vi "AO master control_v2.vi"() -> ()   [LabVIEW 2018]
uses:
  Casao LabVIEW SDK 1.0.5/Haso/Data Haso/Wavefront parameters.ctl
  Casao LabVIEW SDK 1.0.5/Casao/Casao/Casao.ctl
  Casao LabVIEW SDK 1.0.5/Drivers_DPhaseModul/PhaseModul.ctl
  Casao LabVIEW SDK 1.0.5/Casao/CasaoMatrix/CasaoMatrix.ctl
  Casao LabVIEW SDK 1.0.5/Haso/Haso/Haso.ctl
  Casao LabVIEW SDK 1.0.5/Haso/Camera/Camera.ctl
  <vilib>/Utility/error.llb/DialogType.ctl
  Casao LabVIEW SDK 1.0.5/Casao/Casao/Loop prefs.ctl
  Casao LabVIEW SDK 1.0.5/Haso/Data Haso/DataHaso.ctl
  <vilib>/DAQmx/write.llb/DAQmx Write (Digital Bool 1Line 1Point).vi
  <vilib>/Utility/file.llb/Read From Spreadsheet File (DBL).vi
  <vilib>/DAQmx/create/channels.llb/DAQmx Create Channel (DO-Digital Output).vi
  <vilib>/DAQmx/miscellaneous.llb/DAQmx Fill In Error Info.vi
  <vilib>/Utility/file.llb/Write To Spreadsheet File (DBL).vi
panel:
  in  "Phase command 3":path=path "D:/SystemAlignment/system_aberration_20191029.dat"
  in  "Phase command 2":path=path "D:/SystemAlignment/100nm correction.dat"
  in  "Phase command 1":path=path "D:/SystemAlignment/FLAT_MIRAO_0225_01.dat"
  in  "Phase command 0":path=path "D:/SystemAlignment/system_aberration_20191029.dat"
  out "error out 3":errorcluster
  out "error out 2":errorcluster
  out "error out 4":errorcluster
  out "error out":errorcluster
  in  "Control Panel":T1(tab)
  in  "Haso Serial #":T2=7364
  out "Camera Index":T3
  out "Haso Index":T2
  out "Casao Matrix Index":T4
  out "Initialization error":errorcluster
  in  "Matrix Initial":path=path "D:/Data/CM_20191031.aomc"
  out "Mirror Index":T5
  in  "DM Initial":path=path "D:/SystemAlignment/system_aberration_20191029.dat"
  out "Casao Index":T6
  in  "Stage Port":refnum<visa-resource-name>="COM5"
  in  "Flip Mirror Port":tag="Dev1/ao5"
  in  "EMCCD trigger port":tag="Dev1/port0/line0"
  in  "EMCCD fire port":tag="/Dev1/PFI0"
  in  "Laser 2P shutter port":tag="Dev1/port0/line1"
  in  "Laser 488 shutter port":tag="Dev1/port0/line3"
  in  "baud rate (9600)":u32=9600
  in  "Mirao Parameters":path=path "C:/Program Files (x86)/Imagine Optic/Configuration Files/mirao 52-e 0225.xml"
  in  "Haso Exposure (s) Initial":dbl=0.5
  in  "Update DM":bool
  in  "right":bool
  in  "left":bool
  in  "front":bool
  in  "back":bool
  in  "XY step (10=1um)":u16=50
  in  "down":bool
  in  "up":bool
  in  "Z step (10=1um)":dbl=2.0
  in  "stop adjustment":bool
  in  "WideField 488":bool
  in  "Flip Mirror":sgl(ring)=-5.0 items=["EMCCD Camera"=-5, "Wavefront sensor"=1]
  out "Numeric status":dbl
  in  "Two photon":bool
  in  "Offset path":path=path "D:/SystemAlignment/system_aberration_20191029.dat"
  in  "Matrix path":path=path "D:/Data/CM_20191031.aomc"
  in  "Acquisition Mode":T7(ring) caption="Acquistion Mode"
  out "Wavefront after correction":dbl[][](graph) caption="Wavefront"
  out "Wavefront before correction":dbl[][](graph) caption="Wavefront"
  out "output path":path
  in  "Correction":bool
  in  "Slices #":dbl=2.0
  in  "Average Frame #":dbl=1.0
  in  "Offset path 2":path=path "D:/Data/system_aberration_20191029.dat"
  in  "Matrix path 2":path=path "D:/Data/CM_20191031.aomc"
  out "Model Coefficients (µm) before":sgl[](array[numeric])
  in  "Iteration #":u16(ring)=1 items=["1"=1, "2"=2, "3"=3, "4"=4, "5"=5]
  in  "AoExp Time":dbl(ring)=0.5 items=["0.2s"=0.2, "0.5s"=0.5, "1.0s"=1.0, "1.5s"=1.5]
  in  "stop":bool
  out "Camera image":u32[][](graph)
  out "before correction":T8
  out "after correction":T8
  in  "Step size(um)":dbl
  in  "ImExp Time (s)":dbl(ring)=0.1 items=["0.05"=0.05, "0.1"=0.1, "0.2"=0.2, "0.5"=0.5, "1.0"=1.0, "4.0"=4.0, "8.0"=8.0]
  out "Slice now":dbl
  in  "Filter y tilt":bool=TRUE
  in  "Filter x tilt":bool=TRUE
  in  "Curvature filter":bool=TRUE
  out "RMS":dbl
  out "PV":dbl
  out "PV":dbl
  out "RMS":dbl
  in  "Filter y tilt":bool=TRUE
  in  "Filter x tilt":bool=TRUE
  in  "Curvature filter":bool=TRUE
  out "Model Coefficients (µm) after":sgl[](array[numeric])
  out "Shutdown error":errorcluster
  in  "Control Mode":T9(ring)=enum."Parameter Adjustment"
  # "Port connections"
  # "Casao Initialization"
  # "Casao Status"
  # "Sample Stage"
  # "WF switch"
  # "EMCCD: -5"
  # "Wavefront Sensor: 1"
  # "Laser Shutter"
  # "Deformable Mirror"
  # "Wavefront Sensor"
  # "AO correction (Casao)"
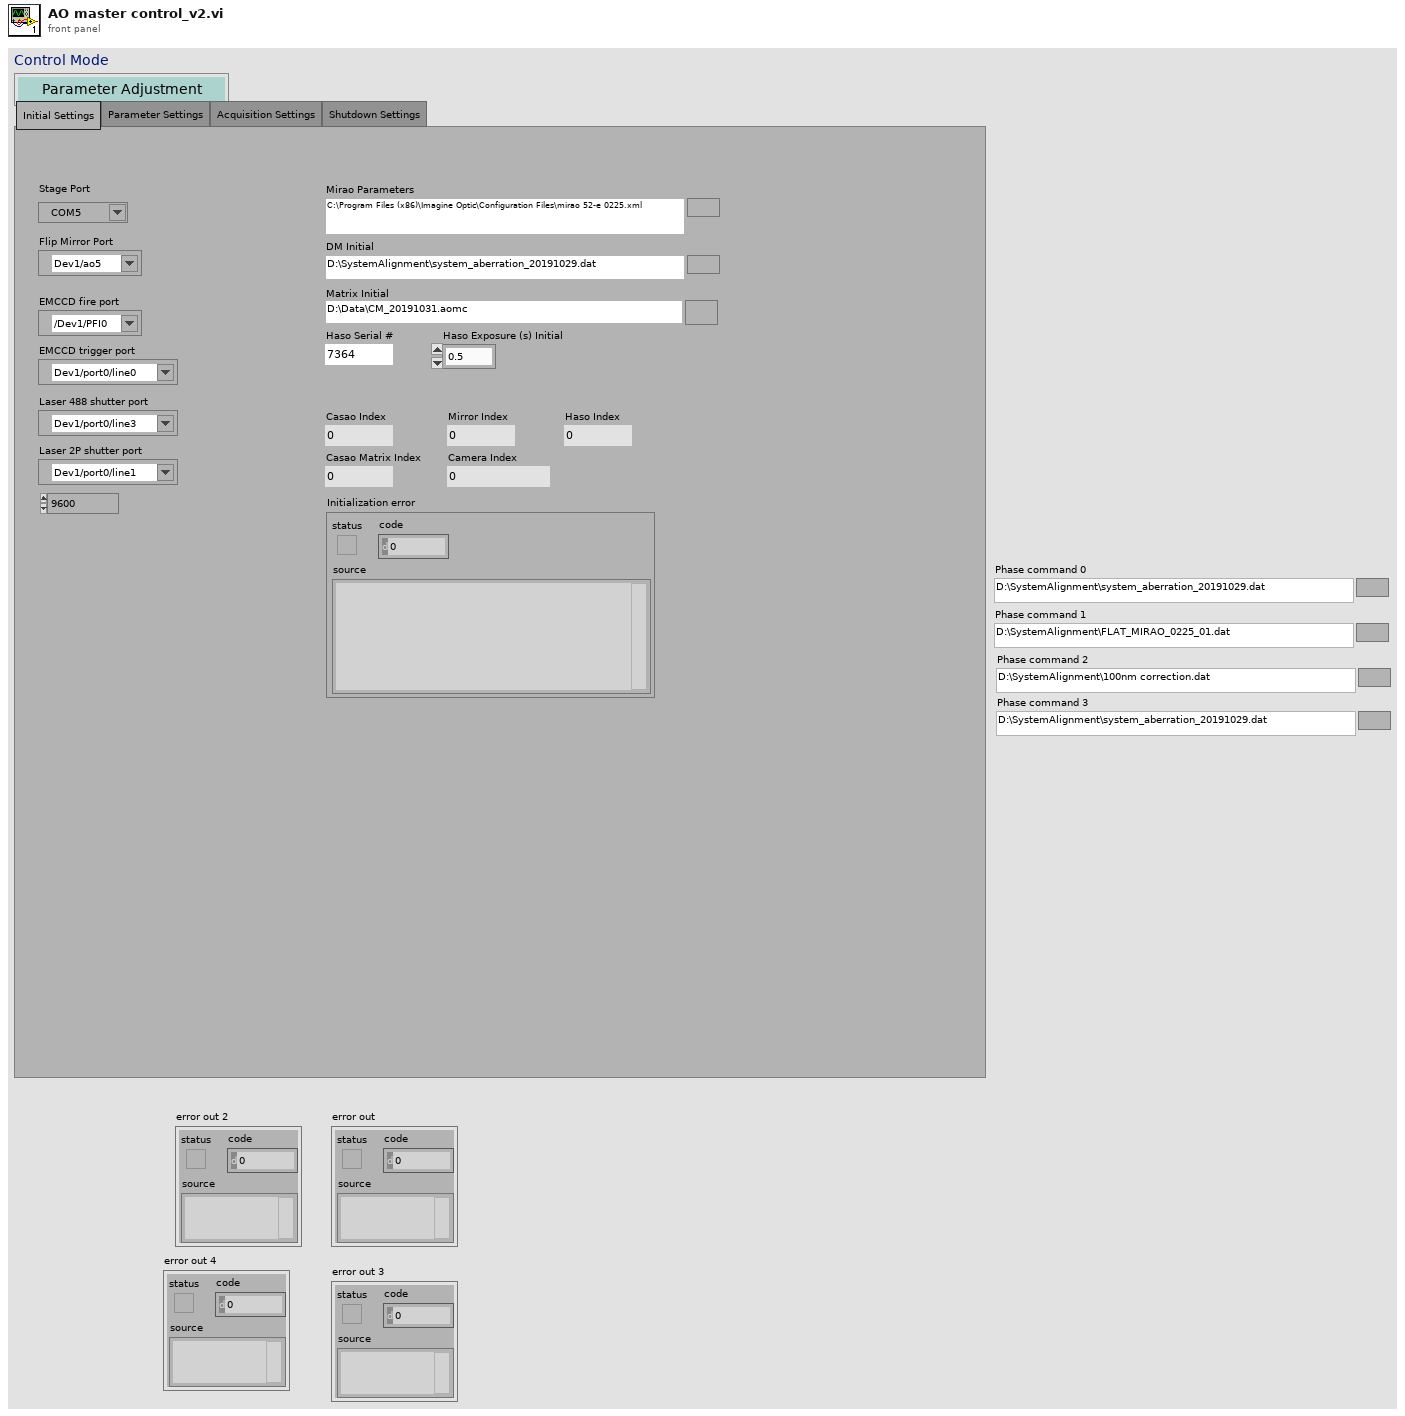
[diagram p1: front panel]
types:
  T1 = enum32{"Initial Settings", "Parameter Settings", "Acquisition Settings", "Shutdown Settings"}
  T2 = typedef "Haso.ctl" = i32
  T3 = typedef "Camera.ctl" = i32
  T4 = typedef "CasaoMatrix.ctl" = i32
  T5 = typedef "PhaseModul.ctl" = i32
  T6 = typedef "Casao.ctl" = i32
  T7 = enum16{"Wide Field", "Wide Field (Phase diversity)", "Two photon"}
  T8 = typedef "Wavefront parameters.ctl" = cluster{"X Tilt (mrad)":sgl, "Y Tilt (mrad)":sgl, "Radius of curvature (mm)":sgl, "X focal point position (mm)":sgl, "Y focal point position (mm)":sgl, "Astigmatism angle (rad)":sgl, "Sagittal focal length (mm)":sgl, "Tangential focal length (mm)":sgl}
  T9 = enum16{"Initialization", "Parameter Adjustment", "Acquisition", "Shut Down"}
  T10 = typedef "Loop prefs.ctl" = cluster{"Filter tilt on measurement (closed loop)":bool, "Correction gain (closed loop)":sgl, "Limit of subapertures off in CGP (%)":sgl, "Limit of saturated actuators (%)":sgl}
  T11 = cluster{"Filtre tilt X":bool, "Filtre tilt Y":bool, "Filtre courbure":bool}
  T12 = typedef "DataHaso.ctl" = i32
  T13 = cluster{"Measurement":T12, "Target":T12, "Manual target":T12}
  T14 = cluster{"Target for tilt":T12, "Target for focus":T12, "Target for all other aberrations":T12}
  T15 = typedef "Camera preferences.ctl" = cluster{"Exposure duration (µs)":u32, "Exposure duration specified (µs)":u32, "Number of summed images":u32, "Trigger type":enum16{"Internal", "TTL", "Software"}, "Trigger event":enum16{"falling", "rising"}, "Remove background image":bool, "Background image":T16, "Path to background image":string, "Auto exposure":bool, "Auto exposure target (%)":sgl, "Auto exposure tolerance (%)":sgl, "Timeout delay (ms)":u32, "Delay after trigger (µs)":i32}
  T16 = typedef "Image Compat.ctl" = cluster{"Signed/unsigned":bool, "Number of bits":T17, "Internal object id":i32, "Internal data id":i32}
  T17 = typedef "Data alignment enum.ctl" = enum16{"8", "16", "32"}
  T18 = typedef "DialogType.ctl" = u16
  T19 = typedef "Reconstruction prefs.ctl" = cluster{"Reconstruction type":enum16{"Modal", "Zonal"}, "Polynomial type":enum16{"Zernike", "Legendre"}, "Modal reconstruction prefs":T20, "Zonal reconstruction prefs":T23}
  T20 = typedef "Modal reconstruction prefs.ctl" = cluster{"Number of coefficients":u32, "Filtered coefficients":u32[], "RMS Zernike normalization":bool, "Matrix inversion method":u16, "Add zonal residual to modal fit ":bool, "Detection prefs":T21}
  T21 = typedef "PupilDetectionPrefs.ctl" = cluster{"Automatic pupil detection":bool, "Central occultation pupil":bool, "Semi-automatic pupil detection (find radius)":bool, "Semi-automatic pupil detection (find center)":bool, "Automatic pupil detection mode":enum16{"Contained", "Containing"}, "Start coordinates":cluster{"Pupil center (Zernike)":T22, "Pupil radius (Zernike)":sgl, "Pupil center (Legendre)":T22, "Pupil halfsize (Legendre)":T22}}
  T22 = typedef "Point2Df.ctl" = cluster{"X":sgl, "Y":sgl}
  T23 = typedef "Zonal reconstruction prefs.ctl" = cluster{"Number of weak iterations":u16, "Number of max iterations":u32, "Residual limit":sgl}
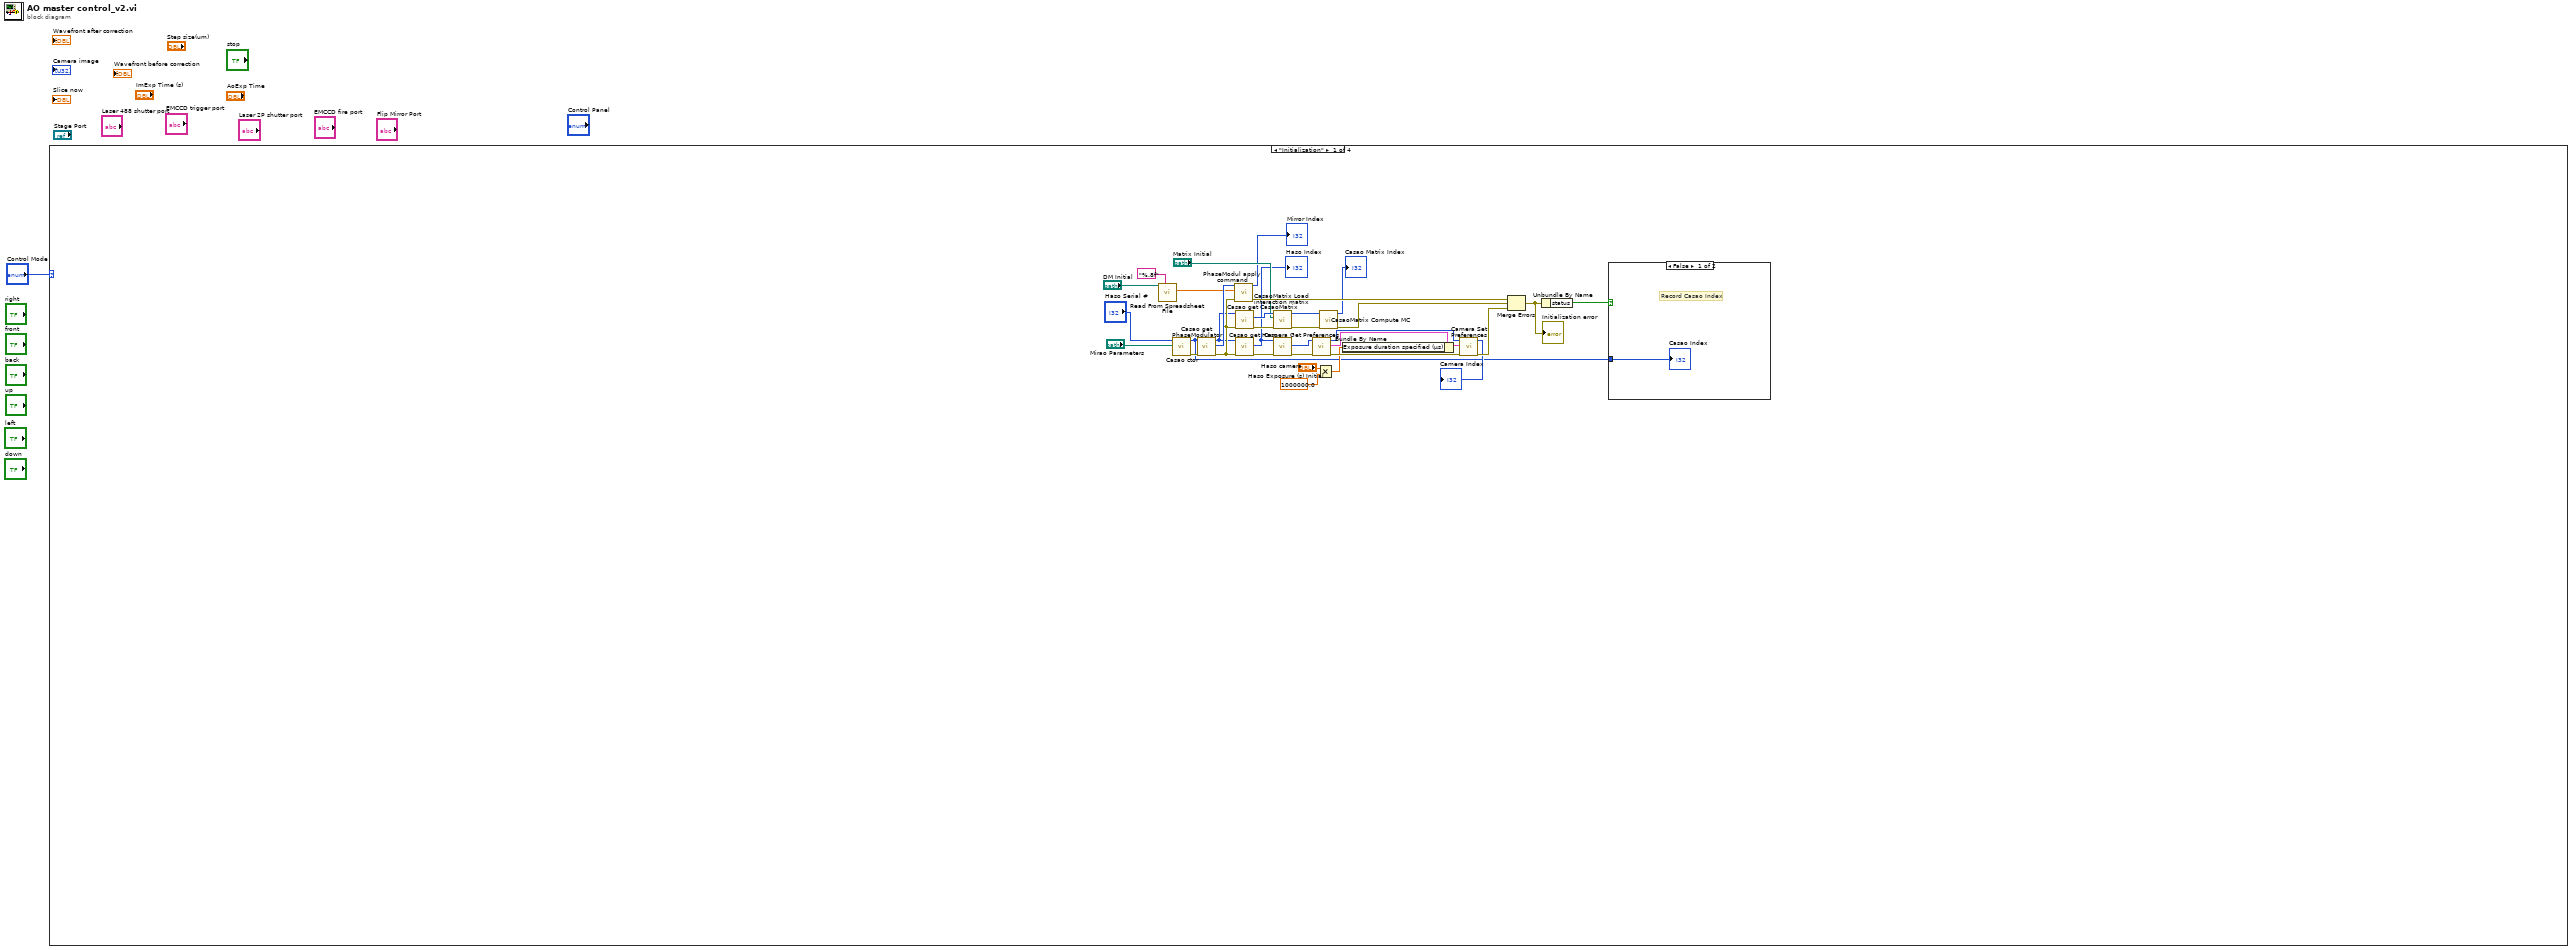
[diagram p0: block diagram]
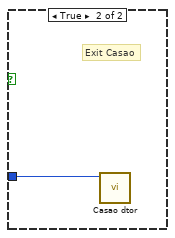
[diagram p2: hidden frame]
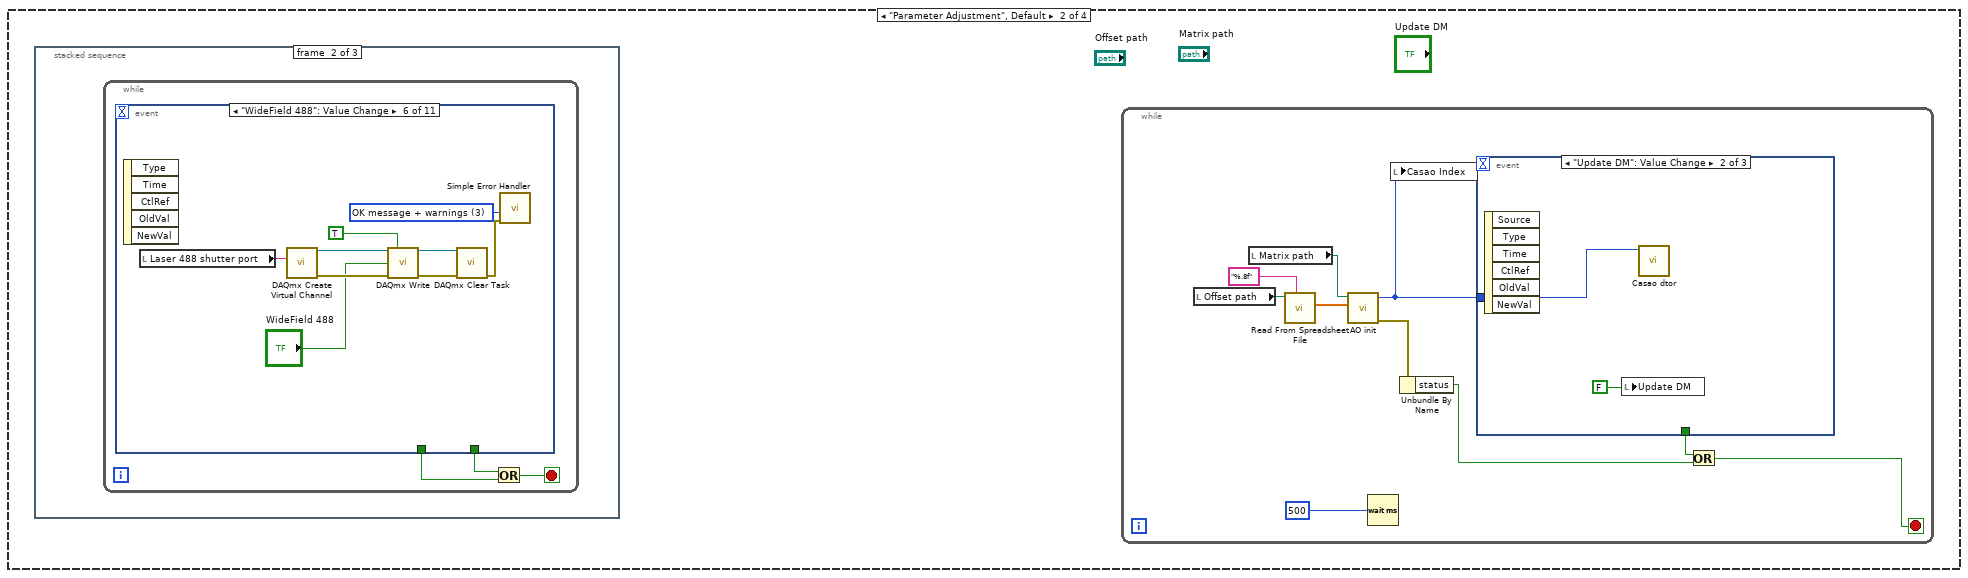
[diagram p3: hidden frame]
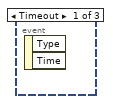
[diagram p4: hidden frame]
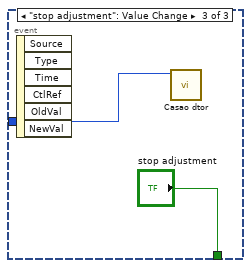
[diagram p5: hidden frame]
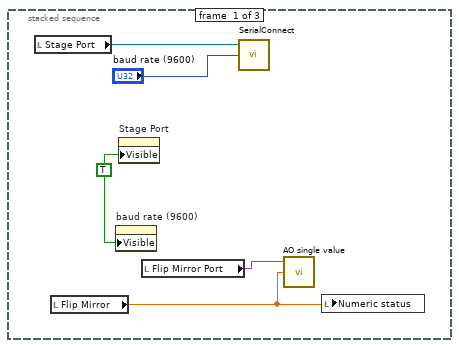
[diagram p6: hidden frame]
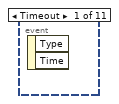
[diagram p7: hidden frame]
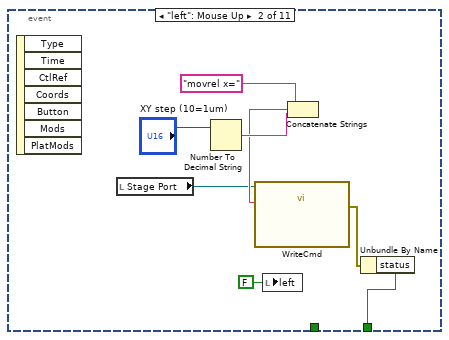
[diagram p8: hidden frame]
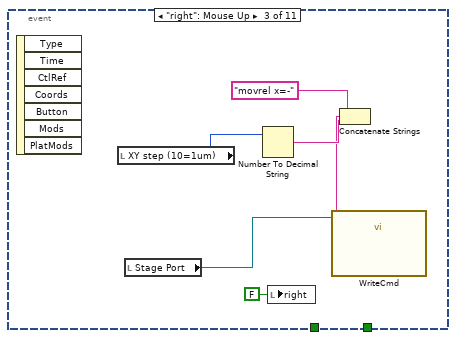
[diagram p9: hidden frame]
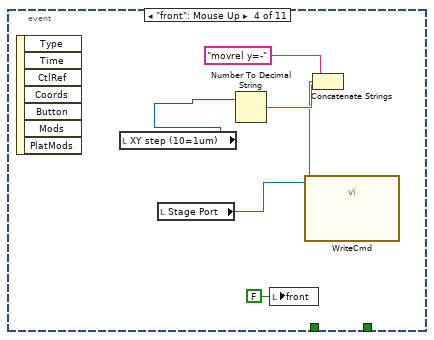
[diagram p10: hidden frame]
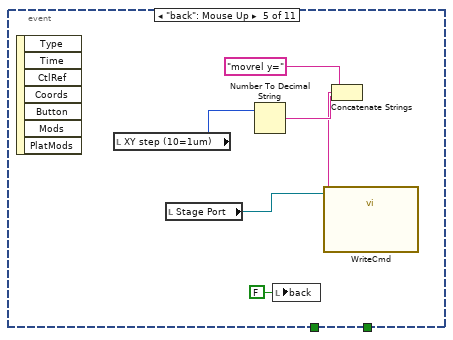
[diagram p11: hidden frame]
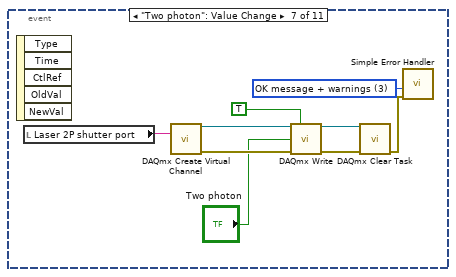
[diagram p12: hidden frame]
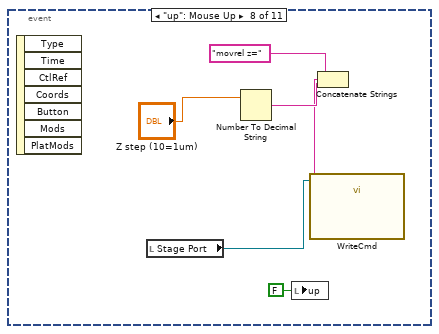
[diagram p13: hidden frame]
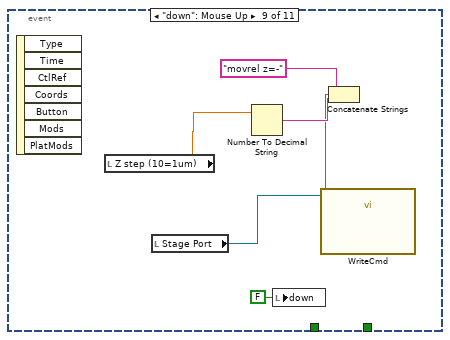
[diagram p14: hidden frame]
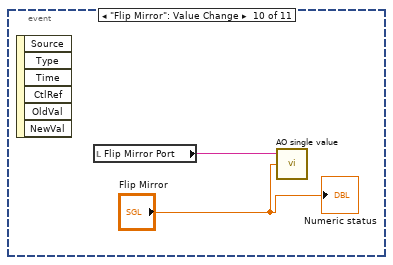
[diagram p15: hidden frame]
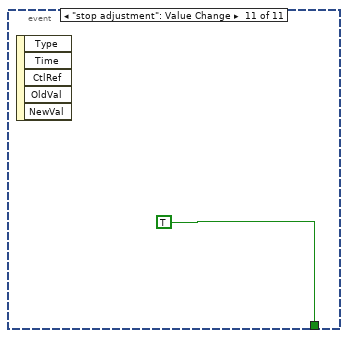
[diagram p16: hidden frame]
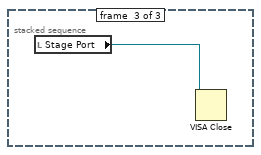
[diagram p17: hidden frame]
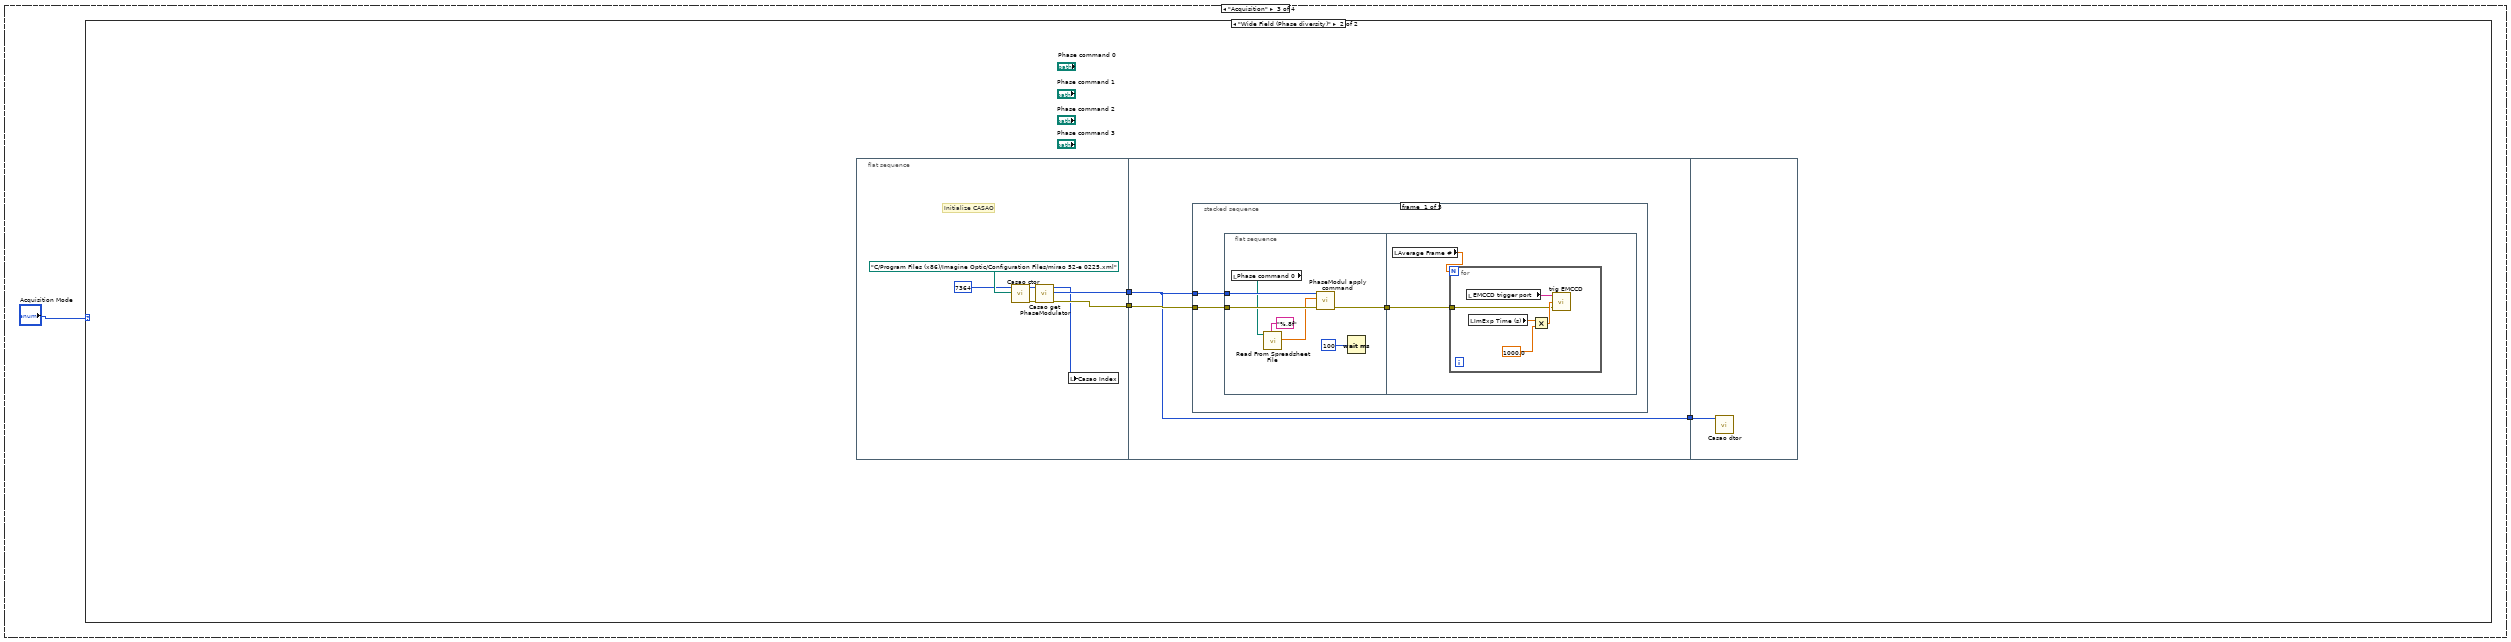
[diagram p18: hidden frame]
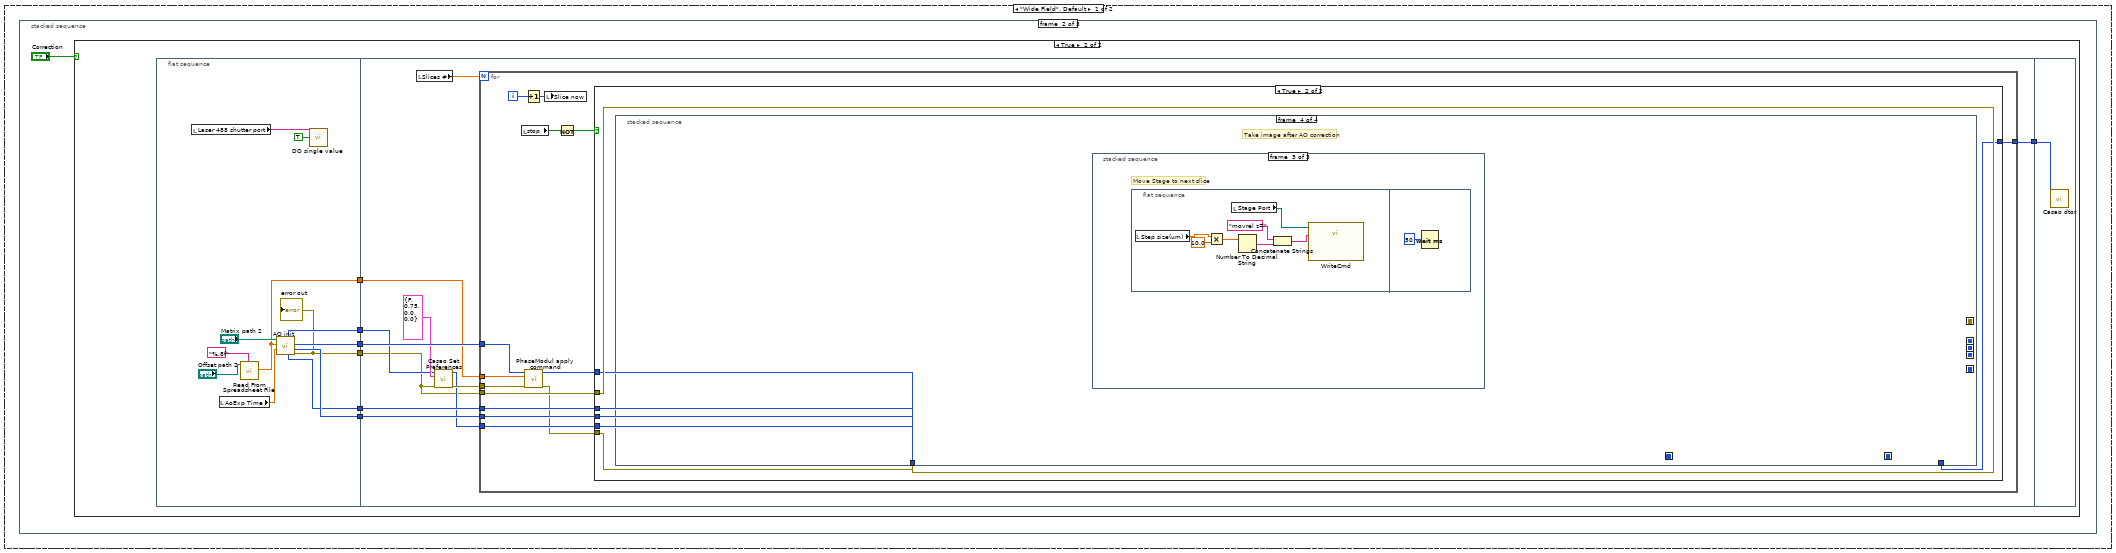
[diagram p19: hidden frame]
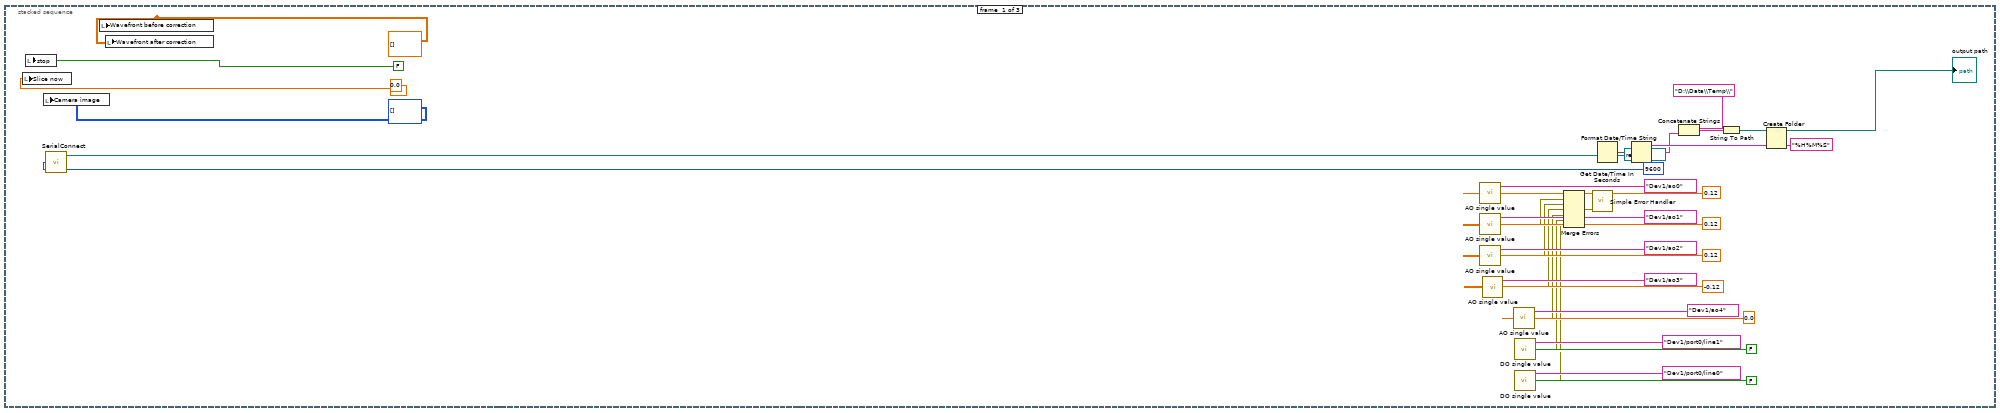
[diagram p20: hidden frame]
diagram:
  n1 = case shown="\"Initialization\"" "Control Mode" {
    frame "Initialization" {
      n2 = call-poly <vilib>:"Read From Spreadsheet File.vi"("format (%.3f)"="%.8f", "file path (dialog if empty)"="DM Initial") -> ("first row"=w10:dbl[])  [unwired: 5 in, 4 out]
      n3 = call "Casao ctor.vi"("Mirror config file path"="Mirao Parameters", "Haso serial number"="Haso Serial #") -> ("error out"=w19:errorcluster, "Casao"=w2:T6)  [unwired: 6 in]
      n4 = call "Casao get PhaseModulator.vi"("error in (no error)"=w19, "Casao"=w2) -> ("error out"=w21:errorcluster, "Mirrror"=w20:T5, "Casao (dup)"=w17:T6)  [unwired: 3 in]
      n5 = call "PhaseModul apply command.vi"("error in (no error)"=w21, "Commands in"=w10, "Mirror"=w20) -> ("error out"=w18:errorcluster, "Mirror (dup)"=→"Mirror Index":T5)  [unwired: 2 in, 1 out]
      n6 = call "Casao get CasaoMatrix.vi"("error in (no error)"=w21, "Casao"=w17) -> ("error out"=w32:errorcluster, "Casao matrix"=w31:T4)  [unwired: 3 in, 1 out]
      n7 = call "Casao get Haso.vi"("error in (no error)"=w21, "Casao"=w17) -> ("error out"=w28:errorcluster, "Haso"=w6:T2)  [unwired: 3 in, 1 out]
      "Haso Index" <- w6
      n8 = call "CasaoMatrix Load interaction matrix.vi"("error in (no error)"=w32, "Path"="Matrix Initial", "Casao matrix"=w31) -> ("error out"=w30:errorcluster, "Casao matrix (dup)"=w29:T4)  [unwired: 1 in, 2 out]
      n9 = call "Haso camera.vi"("error in (no error)"=w28, "Haso"=w6) -> ("error out"=w27:errorcluster, "camera"=w26:T3)  [unwired: 3 in, 1 out]
      n10 = call "Camera Get Preferences.vi"("error in (no error)"=w27, "Camera"=w26) -> ("error out"=w25:errorcluster, "Camera Preferences"=w24:T15, "Camera (dup)"=w23:T3)  [unwired: 3 in]
      n11 = Multiply(x="Haso Exposure (s) Initial", y=1000000.0) -> (x*y=w11:dbl)
      n12 = call "CasaoMatrix Compute MC.vi"("error in (no error)"=w30, "Casao Matrix"=w29) -> ("error out"=w9:errorcluster, "Casao Matrix (dup)"=→"Casao Matrix Index":T4)  [unwired: 4 in]
      n13 = Bundle By Name(cluster=w24, "Exposure duration specified (µs)"=w11) -> (w22:T15)
      n14 = call "Camera Set Preferences.vi"("error in (no error)"=w25, "Camera Preferences"=w22, "Camera"=w23) -> ("error out"=w16:errorcluster, "Camera (dup)"=→"Camera Index":T3)  [unwired: 3 in]
      n15 = Merge Errors(w18, w9, w16) -> (w3:errorcluster)
      "Initialization error" <- w3
      n16 = Unbundle By Name(w3) -> ("status"=w33:bool)
      n17 = case shown="False" w33 {
        tunnel: w2 -> [w36 w37]
        frame False {
          # "Record Casao Index"
          "Casao Index" <- w36
        }
        frame True {
          # "Exit Casao"
          n18 = call "Casao dtor.vi"("Casao"=w37) -> ()  [unwired: 6 in, 1 out]
        }
      }
    }
    frame "Parameter Adjustment", Default {
      n19 = stacked-sequence {
        frame #0 {
          w55 = TRUE ("Visible")
          n20 = local read "Stage Port"() -> (w53:refnum<visa-resource-name>)
          n21 = local read "Flip Mirror"() -> (w54:sgl)
          n22 = property on="baud rate (9600)" class="DigNum (strict)"("Visible"=w55) -> ()  [unwired: 2 in, 2 out]
          n23 = property on="Stage Port" class="VISAName"("Visible"=w55) -> ()  [unwired: 2 in, 2 out]
          n24 = local read "Flip Mirror Port"() -> (w52:tag)
          n25 = call "SerialConnect.vi"("baud rate (9600)"="baud rate (9600)", "VISA resource name"=w53) -> ()  [unwired: 1 in, 3 out]
          n26 = call "AO single value.vi"("data"=w54, "physical channels"=w52) -> ()  [unwired: 1 in, 1 out]
          n27 = local write "Numeric status"(w54) -> ()
        }
        frame #1 {
          n28 = while {
            stop <- w59 stop-if-true
            n29 = event shown="[5] \"WideField 488\": Value Change" {
              selector: _ -> [_ _ _ _ _ _ _ _ _ _ _]
              dyn-events: _ -> [_ _ _ _ _ _ _ _ _ _ _]
              timeout: _ -> [_ _ _ _ _ _ _ _ _ _ _]
              tunnel: [_ _ _ _ _ _ _ _ _ _ TRUE] -> w58
              tunnel: [_ w60 _ _ _ _ _ _ _ _ _] -> w57
              event Timeout {
                n30 = event-data() -> ()  [unwired: 1 in, 2 out]
              }
              event "left": Mouse Up {
                n31 = event-data() -> ()  [unwired: 1 in, 7 out]
                n32 = local read "Stage Port"() -> (w63:refnum<visa-resource-name>)
                n33 = Number To Decimal String(number="XY step (10=1um)") -> (decimal integer string=w65:string)  [unwired: 1 in]
                n34 = local write "left"(FALSE ("left")) -> ()
                n35 = Concatenate Strings("movrel x=", w65) -> (w64:string)
                n36 = call "WriteCmd.vi"("Command"=w64, "VISA resource name"=w63) -> ("error"=w61:errorcluster)  [unwired: 1 in]
                n37 = Unbundle By Name(w61) -> ("status"=w60:bool)
              }
              event "right": Mouse Up {
                n38 = event-data() -> ()  [unwired: 1 in, 7 out]
                n39 = local read "XY step (10=1um)"() -> (w69:u16)
                n40 = local read "Stage Port"() -> (w68:refnum<visa-resource-name>)
                n41 = Number To Decimal String(number=w69) -> (decimal integer string=w72:string)  [unwired: 1 in]
                n42 = local write "right"(FALSE ("right")) -> ()
                n43 = Concatenate Strings("movrel x=-", w72) -> (w71:string)
                n44 = call "WriteCmd.vi"("Command"=w71, "VISA resource name"=w68) -> ()  [unwired: 1 in, 1 out]
              }
              event "front": Mouse Up {
                n45 = event-data() -> ()  [unwired: 1 in, 7 out]
                n46 = local read "XY step (10=1um)"() -> (w74:u16)
                n47 = local read "Stage Port"() -> (w76:refnum<visa-resource-name>)
                n48 = Number To Decimal String(number=w74) -> (decimal integer string=w78:string)  [unwired: 1 in]
                n49 = local write "front"(FALSE ("front")) -> ()
                n50 = Concatenate Strings("movrel y=-", w78) -> (w77:string)
                n51 = call "WriteCmd.vi"("Command"=w77, "VISA resource name"=w76) -> ()  [unwired: 1 in, 1 out]
              }
              event "back": Mouse Up {
                n52 = event-data() -> ()  [unwired: 1 in, 7 out]
                n53 = local read "XY step (10=1um)"() -> (w80:u16)
                n54 = local read "Stage Port"() -> (w82:refnum<visa-resource-name>)
                n55 = Number To Decimal String(number=w80) -> (decimal integer string=w84:string)  [unwired: 1 in]
                n56 = local write "back"(FALSE ("back")) -> ()
                n57 = Concatenate Strings("movrel y=", w84) -> (w83:string)
                n58 = call "WriteCmd.vi"("Command"=w83, "VISA resource name"=w82) -> ()  [unwired: 1 in, 1 out]
              }
              event "WideField 488": Value Change {
                w94 = T18 3 items=["no dialog", "OK message", "continue or stop message", "OK message + warnings", "continue/stop + warnings"] ("type of dialog (OK msg:1)")
                n59 = event-data() -> ()  [unwired: 1 in, 5 out]
                n60 = local read "Laser 488 shutter port"() -> (w86:tag)
                n61 = call-poly <vilib>:"DAQmx Create Virtual Channel.vi"("lines"=w86) -> ("task out"=w90:refnum<k21>, "error out"=w91:errorcluster)  [unwired: 13 in]
                n62 = call-poly <vilib>:"DAQmx Write.vi"("task/channels in"=w90, "auto start"=TRUE, "data"="WideField 488", "error in"=w91) -> ("task out"=w89:refnum<k21>, "error out"=w88:errorcluster)  [unwired: 9 in, 1 out]
                n63 = call <vilib>:"DAQmx Clear Task.vi"("task in"=w89, "error in"=w88) -> ("error out"=w93:errorcluster)  [unwired: 13 in]
                n64 = call <vilib>:"Simple Error Handler.vi"("type of dialog (OK msg:1)"=w94, "error in (no error)"=w93) -> ()  [unwired: 3 in, 5 out]
              }
              event "Two photon": Value Change {
                w103 = T18 3 items=["no dialog", "OK message", "continue or stop message", "OK message + warnings", "continue/stop + warnings"] ("type of dialog (OK msg:1)")
                n65 = event-data() -> ()  [unwired: 1 in, 5 out]
                n66 = local read "Laser 2P shutter port"() -> (w95:tag)
                n67 = call-poly <vilib>:"DAQmx Create Virtual Channel.vi"("lines"=w95) -> ("task out"=w99:refnum<k21>, "error out"=w100:errorcluster)  [unwired: 13 in]
                n68 = call-poly <vilib>:"DAQmx Write.vi"("task/channels in"=w99, "auto start"=TRUE, "data"="Two photon", "error in"=w100) -> ("task out"=w98:refnum<k21>, "error out"=w97:errorcluster)  [unwired: 9 in, 1 out]
                n69 = call <vilib>:"DAQmx Clear Task.vi"("task in"=w98, "error in"=w97) -> ("error out"=w102:errorcluster)  [unwired: 13 in]
                n70 = call <vilib>:"Simple Error Handler.vi"("type of dialog (OK msg:1)"=w103, "error in (no error)"=w102) -> ()  [unwired: 3 in, 5 out]
              }
              event "up": Mouse Up {
                n71 = event-data() -> ()  [unwired: 1 in, 7 out]
                n72 = local read "Stage Port"() -> (w106:refnum<visa-resource-name>)
                n73 = Number To Decimal String(number="Z step (10=1um)") -> (decimal integer string=w108:string)  [unwired: 1 in]
                n74 = local write "up"(FALSE ("up")) -> ()
                n75 = Concatenate Strings("movrel z=", w108) -> (w107:string)
                n76 = call "WriteCmd.vi"("Command"=w107, "VISA resource name"=w106) -> ()  [unwired: 1 in, 1 out]
              }
              event "down": Mouse Up {
                n77 = event-data() -> ()  [unwired: 1 in, 7 out]
                n78 = local read "Z step (10=1um)"() -> (w110:dbl)
                n79 = local read "Stage Port"() -> (w112:refnum<visa-resource-name>)
                n80 = Number To Decimal String(number=w110) -> (decimal integer string=w114:string)  [unwired: 1 in]
                n81 = local write "down"(FALSE ("down")) -> ()
                n82 = Concatenate Strings("movrel z=-", w114) -> (w113:string)
                n83 = call "WriteCmd.vi"("Command"=w113, "VISA resource name"=w112) -> ()  [unwired: 1 in, 1 out]
              }
              event "Flip Mirror": Value Change {
                n84 = event-data() -> ()  [unwired: 1 in, 6 out]
                n85 = local read "Flip Mirror Port"() -> (w116:tag)
                n86 = call "AO single value.vi"("data"="Flip Mirror", "physical channels"=w116) -> ()  [unwired: 1 in, 1 out]
                "Numeric status" <- "Flip Mirror"
              }
              event "stop adjustment": Value Change {
                n87 = event-data() -> ()  [unwired: 1 in, 5 out]
              }
            }
            n88 = Or(x=w57, y=w58) -> (x .or. y?=w59:bool)
          }
        }
        frame #2 {
          n89 = local read "Stage Port"() -> (w119:refnum<visa-resource-name>)
          n90 = VISA Close(VISA resource name=w119) -> ()  [unwired: 1 in, 1 out]
        }
      }
      n91 = while {
        stop <- w47 stop-if-true
        n92 = local read "Offset path"() -> (w44:path)
        n93 = local read "Matrix path"() -> (w43:path)
        n94 = call-poly <vilib>:"Read From Spreadsheet File.vi"("format (%.3f)"="%.8f", "file path (dialog if empty)"=w44) -> ("first row"=w45:dbl[])  [unwired: 5 in, 4 out]
        n95 = call "AO init.vi"("Commands in"=w45, "Matrix path"=w43) -> ("error out"=w41:errorcluster, "Casao"=w38:T6)  [unwired: 4 in, 4 out]
        n96 = Wait (ms)(milliseconds to wait=500) -> ()  [unwired: 1 out]
        n97 = local write "Casao Index"(w38) -> ()
        n98 = Unbundle By Name(w41) -> ("status"=w40:bool)
        n99 = event shown="[1] \"Update DM\": Value Change" {
          selector: _ -> [_ _ _]
          dyn-events: _ -> [_ _ _]
          timeout: _ -> [_ _ _]
          tunnel: [_ _ "stop adjustment"] -> w39
          tunnel: w38 -> [_ w49 w51]
          event Timeout {
            n100 = event-data() -> ()  [unwired: 1 in, 2 out]
          }
          event "Update DM": Value Change {
            n101 = event-data() -> ()  [unwired: 1 in, 6 out]
            n102 = local write "Update DM"(FALSE) -> ()
            n103 = call "Casao dtor.vi"("Casao"=w49) -> ()  [unwired: 6 in, 1 out]
          }
          event "stop adjustment": Value Change {
            n104 = event-data() -> ()  [unwired: 1 in, 6 out]
            n105 = call "Casao dtor.vi"("Casao"=w51) -> ()  [unwired: 6 in, 1 out]
          }
        }
        n106 = Or(x=w39, y=w40) -> (x .or. y?=w47:bool)
      }
    }
    frame "Acquisition" {
      n107 = case shown="\"Wide Field (Phase diversity)\"" "Acquisition Mode" {
        frame "Wide Field", Default {
          n108 = stacked-sequence {
            frame #0 {
              w123 = dbl[][] [] ("before correction")
              n109 = local write "Slice now"(0.0 ("Slice now")) -> ()
              n110 = local write "stop"(FALSE ("stop")) -> ()
              n111 = local write "Camera image"(u32[][] [] ("Camera image")) -> ()
              n112 = call "SerialConnect.vi"("baud rate (9600)"=u32 9600, "VISA resource name"=refnum<visa-resource-name> "COM1") -> ()  [unwired: 1 in, 3 out]
              n113 = local write "Wavefront before correction"(w123) -> ()
              n114 = local write "Wavefront after correction"(w123) -> ()
              n115 = call "AO single value.vi"("data"=0.12, "physical channels"=tag "Dev1/ao0") -> ("error out"=w139:errorcluster)  [unwired: 1 in]
              n116 = call "AO single value.vi"("data"=0.12, "physical channels"=tag "Dev1/ao1") -> ("error out"=w138:errorcluster)  [unwired: 1 in]
              n117 = call "AO single value.vi"("data"=0.12, "physical channels"=tag "Dev1/ao2") -> ("error out"=w137:errorcluster)  [unwired: 1 in]
              n118 = call "AO single value.vi"("data"=-0.12, "physical channels"=tag "Dev1/ao3") -> ("error out"=w136:errorcluster)  [unwired: 1 in]
              n119 = call "AO single value.vi"("data"=0.0, "physical channels"=tag "Dev1/ao4") -> ("error out"=w135:errorcluster)  [unwired: 1 in]
              n120 = call "DO single value.vi"("data"=FALSE, "lines"=tag "Dev1/port0/line1") -> ("error out"=w134:errorcluster)  [unwired: 1 in]
              n121 = call "DO single value.vi"("data"=FALSE, "lines"=tag "Dev1/port0/line0") -> ("error out"=w132:errorcluster)  [unwired: 1 in]
              n122 = Merge Errors(w139, w138, w137, w136, w135, w134, w132) -> (w133:errorcluster)
              n123 = call <vilib>:"Simple Error Handler.vi"("error in (no error)"=w133) -> ()  [unwired: 4 in, 5 out]
              n124 = Get Date/Time In Seconds() -> (seconds since 1Jan1904=w130:timestamp)
              n125 = Format Date/Time String(time format string (%c)="%H%M%S", seconds (now)=w130) -> (date/time string=w127:string)  [unwired: 1 in]
              n126 = Concatenate Strings("D:\\Data\\Temp\\" ("string"), w127) -> (w126:string)
              n127 = String To Path(string=w126) -> (path=w125:path)
              n128 = Create Folder(path (use dialog)=w125) -> (created path=→"output path":path)  [unwired: 2 in, 2 out]
            }
            frame #1 {
              n129 = case shown="True" "Correction" {
                frame False {
                  n130 = flat-sequence {
                    frame #0 {
                      n131 = local read "Laser 488 shutter port"() -> (w157:tag)
                      n132 = call "DO single value.vi"("data"=TRUE, "lines"=w157) -> ()  [unwired: 1 in, 1 out]
                    }
                    frame #1 {
                      n133 = for {
                        N: "Slices #" -> [_]
                        i -> [w163]
                        n134 = local read "stop"() -> (w161:bool)
                        n135 = Not(x=w161) -> (.not. x?=w160:bool)
                        n136 = Increment(x=w163) -> (x+1=w162:i32)
                        n137 = case shown="True" w160 {
                          tunnel: w162 -> [_ w164]
                          frame False {
                          }
                          frame True {
                            n138 = local write "Slice now"(w164) -> ()
                            n139 = stacked-sequence {
                              frame #0 {
                                n140 = for {
                                N: "Average Frame #" -> [_]
                                n141 = local read "stop"() -> (w166:bool)
                                n142 = Not(x=w166) -> (.not. x?=w167:bool)
                                n143 = case shown="True" w167 {
                                frame False {
                                }
                                frame True {
                                n144 = local read "EMCCD trigger port"() -> (w169:tag)
                                n145 = local read "ImExp Time (s)"() -> (w168:dbl)
                                n146 = Multiply(x=w168, y=1000.0) -> (x*y=w170:dbl)
                                n147 = call "trig EMCCD.vi"("exp time (ms)"=w170, "lines"=w169) -> ()  [unwired: 1 in, 1 out]
                                }
                                }
                                }
                              }
                              frame #1 {
                                n148 = local read "Step size(um)"() -> (w173:dbl)
                                n149 = Multiply(x=w173, y=10.0) -> (x*y=w174:dbl)
                                n150 = Number To Decimal String(number=w174) -> (decimal integer string=w177:string)  [unwired: 1 in]
                                n151 = Concatenate Strings("movrel z=", w177) -> (w176:string)
                                n152 = local read "Stage Port"() -> (w172:refnum<visa-resource-name>)
                                n153 = call "WriteCmd.vi"("Command"=w176, "VISA resource name"=w172) -> ()  [unwired: 1 in, 1 out]
                              }
                              frame #2 {
                                n154 = Wait (ms)(milliseconds to wait=u32 100) -> ()  [unwired: 1 out]
                              }
                            }
                          }
                        }
                      }
                    }
                    frame #2 {
                      n155 = local read "Laser 488 shutter port"() -> (w180:tag)
                      n156 = call "DO single value.vi"("data"=FALSE, "lines"=w180) -> ()  [unwired: 1 in, 1 out]
                    }
                  }
                }
                frame True {
                  n157 = flat-sequence {
                    tunnel: [w195] -> w188
                    tunnel: [w194] -> w187
                    tunnel: [w190] -> w186
                    tunnel: [w193] -> w185
                    tunnel: [w192] -> w183
                    tunnel: [w191] -> w182
                    tunnel: w188 -> [w210]
                    tunnel: w187 -> [w209]
                    tunnel: w186 -> [w201]
                    tunnel: w185 -> [w204]
                    tunnel: [w208] -> w184
                    tunnel: w183 -> [w207]
                    tunnel: w182 -> [w202]
                    tunnel: w184 -> [w563]
                    frame #0 {
                      n158 = local read "Laser 488 shutter port"() -> (w189:tag)
                      n159 = local read "AoExp Time"() -> (w196:dbl)
                      n160 = call-poly <vilib>:"Read From Spreadsheet File.vi"("format (%.3f)"="%.8f", "file path (dialog if empty)"="Offset path 2") -> ("first row"=w191:dbl[])  [unwired: 5 in, 4 out]
                      n161 = call "AO init.vi"("Exposure duration specified (s)"=w196, "Commands in"=w191, "Matrix path"="Matrix path 2") -> ("error out"=w190:errorcluster, "Camera"=w195:T3, "Mirror"=w192:T5, "Haso"=w194:T2, "Casao"=w193:T6)  [unwired: 3 in, 1 out]
                      "error out" <- w190
                      n162 = call "DO single value.vi"("data"=TRUE, "lines"=w189) -> ()  [unwired: 1 in, 1 out]
                    }
                    frame #1 {
                      n163 = local read "Slices #"() -> (w211:dbl)
                      n164 = call "Casao Set Preferences.vi"("error in (no error)"=w201, "Loop preferences"=T10 {"Filter tilt on measurement (closed loop)"=FALSE, "Correction gain (closed loop)"=0.75, "Limit of subapertures off in CGP (%)"=0.0, "Limit of saturated actuators (%)"=0.0}, "Casao"=w204) -> ("error out"=w205:errorcluster, "Casao (dup)"=w203:T6)  [unwired: 3 in]
                      n165 = for {
                        N: w211 -> [_]
                        tunnel: w201 -> [w225]
                        tunnel: w210 -> [w224]
                        tunnel: w209 -> [w223]
                        tunnel: w205 -> [w214]
                        tunnel: [w222] -> w208
                        tunnel: w207 -> [w216]
                        tunnel: w203 -> [w221]
                        tunnel: w202 -> [w217]
                        i -> [w218]
                        n166 = local read "stop"() -> (w220:bool)
                        n167 = Increment(x=w218) -> (x+1=w212:i32)
                        n168 = call "PhaseModul apply command.vi"("error in (no error)"=w214, "Commands in"=w217, "Mirror"=w216) -> ("error out"=w213:errorcluster, "Mirror (dup)"=w215:T5)  [unwired: 2 in, 1 out]
                        n169 = local write "Slice now"(w212) -> ()
                        n170 = Not(x=w220) -> (.not. x?=w219:bool)
                        n171 = case shown="True" w219 {
                          tunnel: w225 -> [_ w233]
                          tunnel: w224 -> [_ w232]
                          tunnel: w223 -> [_ w231]
                          tunnel: w213 -> [_ w230]
                          tunnel: [w226 w227] -> w222
                          tunnel: w215 -> [_ w229]
                          tunnel: w221 -> [w226 w228]
                          frame False {
                          }
                          frame True {
                            n172 = stacked-sequence {
                              seq-local: [w239 _ _ _] -> [_ w278 _ _]
                              seq-local: [w238 _ _ _] -> [_ w277 _ _]
                              seq-local: [w237 _ _ _] -> [_ w276 _ _]
                              seq-local: [w236 _ _ _] -> [_ w274 _ _]
                              seq-local: [w235 _ _ _] -> [_ w262 _ _]
                              seq-local: [w234 _ _ _] -> [_ w275 _ _]
                              seq-local: [_ w273 _ _] -> [_ _ w374 _]
                              seq-local: [_ w272 _ _] -> [_ _ w373 _]
                              seq-local: [_ w268 _ _] -> [_ _ w372 _]
                              seq-local: [_ w266 _ _] -> [_ _ w371 _]
                              seq-local: [_ w264 _ _] -> [_ _ w370 _]
                              seq-local: [_ w261 _ _] -> [_ _ w369 _]
                              seq-local: [_ w259 _ _] -> [_ _ w368 _]
                              tunnel: w233 -> [w239 _ _ _]
                              tunnel: w232 -> [w238 _ _ _]
                              tunnel: w231 -> [w237 _ _ _]
                              tunnel: w230 -> [w236 _ _ _]
                              tunnel: w229 -> [w235 _ _ _]
                              tunnel: w228 -> [w234 _ _ _]
                              tunnel: [_ _ w367 _] -> w227
                              frame #0 {
                                # "Take images before AO correction"
                                n173 = stacked-sequence {
                                frame #0 {
                                # "Set detection to EMCCD"
                                n174 = local read "Flip Mirror Port"() -> (w240:tag)
                                n175 = Wait (ms)(milliseconds to wait=u32 100) -> ()  [unwired: 1 out]
                                n176 = call "AO single value.vi"("data"=-5.0, "physical channels"=w240) -> ()  [unwired: 1 in, 1 out]
                                }
                                frame #1 {
                                # "Take image frames"
                                n177 = local read "Average Frame #"() -> (w243:dbl)
                                n178 = for {
                                N: w243 -> [_]
                                n179 = local read "stop"() -> (w244:bool)
                                n180 = Not(x=w244) -> (.not. x?=w245:bool)
                                n181 = case shown="False" w245 {
                                frame False {
                                }
                                frame True {
                                # "EMCCD camera trigger"
                                n182 = local read "EMCCD trigger port"() -> (w247:tag)
                                n183 = local read "ImExp Time (s)"() -> (w246:dbl)
                                n184 = Multiply(x=w246, y=1000.0) -> (x*y=w248:dbl)
                                n185 = call "trig EMCCD.vi"("exp time (ms)"=w248, "lines"=w247) -> ()  [unwired: 1 in, 1 out]
                                }
                                }
                                }
                                }
                                frame #2 {
                                # "Set detection to Wavefront Sensor"
                                n186 = local read "Flip Mirror Port"() -> (w250:tag)
                                n187 = call "AO single value.vi"("data"=1.0, "physical channels"=w250) -> ("error out"=→"error out 4":errorcluster)  [unwired: 1 in]
                                }
                                }
                              }
                              frame #1 {
                                # "Measure aberration"
                                n188 = flat-sequence {
                                tunnel: [w279] -> w258
                                tunnel: [w284] -> w257
                                tunnel: [w280] -> w256
                                tunnel: [w283] -> w255
                                tunnel: [w282] -> w254
                                tunnel: [w281] -> w253
                                tunnel: w278 -> [w285]
                                tunnel: w277 -> [w286]
                                tunnel: w276 -> [w279]
                                tunnel: w275 -> [w283]
                                tunnel: w274 -> [w282]
                                tunnel: w262 -> [w281]
                                tunnel: w256 -> [w359]
                                tunnel: w257 -> [w326]
                                tunnel: w258 -> [w327]
                                tunnel: w255 -> [w347]
                                tunnel: w254 -> [w346]
                                tunnel: [w330] -> w271
                                tunnel: [w329] -> w270
                                tunnel: [w328] -> w269
                                tunnel: [w327] -> w267
                                tunnel: [w326] -> w265
                                tunnel: [w325] -> w263
                                tunnel: w253 -> [w324]
                                tunnel: [w324] -> w260
                                tunnel: [w299] -> w259
                                tunnel: [w365] -> w272
                                tunnel: [w366] -> w273
                                tunnel: w271 -> [w366]
                                tunnel: w270 -> [w365]
                                tunnel: w269 -> [w364]
                                tunnel: [w363] -> w268
                                tunnel: w267 -> [w363]
                                tunnel: [w362] -> w266
                                tunnel: w265 -> [w362]
                                tunnel: [w361] -> w264
                                tunnel: w263 -> [w361]
                                tunnel: [w360] -> w261
                                tunnel: w260 -> [w360]
                                frame #0 {
                                n189 = call "Camera Start.vi"("error in (no error)"=w285, "camera"=w286) -> ("error out"=w280:errorcluster, "camera (dup)"=w284:T3)  [unwired: 4 in]
                                "error out 2" <- w280
                                }
                                frame #1 {
                                n190 = call "Camera Get image.vi"("error in (no error)"=w359, "camera"=w326) -> ("error out"=w343:errorcluster, "Image"=w344:T16, "camera (dup)"=w345:T3)  [unwired: 3 in]
                                n191 = call "Camera Stop.vi"("error in (no error)"=w343, "camera"=w345) -> ()  [unwired: 4 in, 2 out]
                                n192 = call "Image get data.vi"("error in (no error)"=w343, "Image Compat"=w344) -> ("error out"=w292:errorcluster, "Array"=w289:u32[][], "Image Compat (dup)"=w335:T16)  [unwired: 3 in]
                                "error out 3" <- w292
                                n193 = local write "Camera image"(w289) -> ()
                                n194 = call "Haso compute slopes.vi"("error in (no error)"=w292, "Image Compat"=w335, "Haso"=w327) -> ("error out"=w297:errorcluster, "Data Haso"=w301:T12)  [unwired: 1 in, 2 out]
                                n195 = call "DataHaso ctor copie.vi"("error in (no error)"=w297, "DataHaso"=w301) -> ("error out"=w296:errorcluster, "new DataHaso"=w299:T12, "DataHaso (dup)"=w298:T12)  [unwired: 3 in]
                                n196 = call "DataHaso get reconstruction prefs.vi"("error in (no error)"=w296, "Data Haso"=w298) -> ("error out"=w312:errorcluster, "Reconstruction Preferences"=w308:T19, "Data Haso (dup)"=w311:T12)  [unwired: 3 in]
                                n197 = Bundle By Name(cluster=w308, "Reconstruction type"=enum16{"Modal", "Zonal"}."Modal", "Polynomial type"=enum16{"Zernike", "Legendre"}."Zernike", "Modal reconstruction prefs.Number of coefficients"=u32 32) -> (w307:T19)
                                n198 = call "DataHaso set reconstruction prefs.vi"("error in (no error)"=w312, "Reconstruction Preferences"=w307, "Data Haso"=w311) -> ("error out"=w309:errorcluster, "Data Haso (dup)"=w310:T12)  [unwired: 3 in]
                                n199 = call "DataHaso get modal coefficients.vi"("error in (no error)"=w309, "Data Haso"=w310) -> ("error out"=w302:errorcluster, "Coefficients (µm)"=w313:sgl[], "Data Haso (dup)"=w303:T12)  [unwired: 3 in]
                                "Model Coefficients (µm) before" <- w313
                                n200 = call "DataHaso parameters.vi"("error in (no error)"=w302, "Data Haso"=w303) -> ("error out"=w341:errorcluster, "Parameters"=w320:T8, "Data Haso (dup)"=w342:T12)  [unwired: 3 in]
                                "before correction" <- w320
                                n201 = Cluster To Array(cluster=w320) -> (array=w321:sgl[])
                                n202 = Bundle By Name(cluster=T11 {"Filtre tilt X"=TRUE, "Filtre tilt Y"=FALSE, "Filtre courbure"=FALSE} ("Filtre"), "Filtre tilt X"="Filter x tilt", "Filtre tilt Y"="Filter y tilt", "Filtre courbure"="Curvature filter") -> (w290:T11)
                                n203 = call "DataHaso filter tilt or curvature.vi"("error in (no error)"=w341, "Filter (default: all true)"=w290, "Data Haso"=w342) -> ("error out"=w339:errorcluster, "Data Haso (dup)"=w340:T12)  [unwired: 3 in]
                                n204 = call "DataHaso phase.vi"("error in (no error)"=w339, "Data Haso"=w340) -> ("error out"=w338:errorcluster, "Phase (µm)"=w291:i32, "Data Haso (dup)"=w300:T12)  [unwired: 3 in]
                                n205 = control-ref of="Wavefront before correction"() -> (w287:refnum<vi>)
                                n206 = local read "Slice now"() -> (w288:dbl)
                                n207 = call "Formatter Intensity Graph.vi"("error in (no error)"=w338, "Intensity Graph"=w287, "Surface with pupil"=w291) -> ("error out"=w336:errorcluster, "Surface with pupil (dup)"=w337:i32)  [unwired: 2 in, 1 out]
                                n208 = Number To Decimal String(number=w288) -> (decimal integer string=w316:string)  [unwired: 1 in]
                                n209 = call "Surface with pupil get stats.vi"("error in (no error)"=w336, "Surface Avec Pupille"=w337) -> ("error out"=w325:errorcluster, "PV"=w323:sgl, "RMS"=w322:dbl)  [unwired: 2 in, 1 out]
                                "PV" <- w323
                                "RMS" <- w322
                                n210 = local read "output path"() -> (w295:path)
                                n211 = Concatenate Strings("before_slice", w316, ".dat") -> (w294:string)
                                n212 = Build Array (concatenate)(w323, w322, w321, w313) -> (w319:dbl[])
                                n213 = Build Path(base path=w295, name or relative path=w294) -> (appended path=w293:path)
                                n214 = call-poly <vilib>:"Write To Spreadsheet File.vi"("transpose? (no:F)"=TRUE, "format (%.3f)"="%.6f", "1D data"=w319, "file path (dialog if empty)"=w293) -> ()  [unwired: 4 in, 1 out]
                                n215 = Merge Errors(w325, w346) -> (w354:errorcluster)
                                n216 = Bundle By Name(cluster=T14 {"Target for tilt"=0, "Target for focus"=0, "Target for all other aberrations"=0} ("References"), "Target for tilt"=w299, "Target for focus"=w299) -> (w357:T14)
                                n217 = call "DataHaso ctor copie.vi"("error in (no error)"=w354, "DataHaso"=w300) -> ("error out"=w356:errorcluster, "new DataHaso"=w355:T12)  [unwired: 3 in, 1 out]
                                n218 = call "Casao Compute target.vi"("error in (no error)"=w356, "Targets"=w357, "DataHaso"=w355, "Casao"=w347) -> ("error out"=w352:errorcluster, "DataHaso (dup)"=w328:T12, "Casao (dup)"=w353:T6)  [unwired: 1 out]
                                n219 = Bundle By Name(cluster=T13 {"Measurement"=0, "Target"=0, "Manual target"=0} ("Slopes"), "Measurement"=w300, "Target"=w328) -> (w351:T13)
                                n220 = call "Casao get correction commands.vi"("Casao"=w353, "Slopes"=w351, "error in (no error)"=w352) -> ("Casao (dup)"=w330:T6, "Commands"=w348:sgl[], "error out"=w349:errorcluster)  [unwired: 2 in, 2 out]
                                n221 = call "PhaseModul apply command.vi"("error in (no error)"=w349, "Commands in"=w348, "Mirror"=w324) -> ("error out"=w329:errorcluster)  [unwired: 2 in, 2 out]
                                }
                                frame #2 {
                                n222 = call "DataHaso dtor.vi"("Data Haso"=w364) -> ()  [unwired: 6 in, 1 out]
                                }
                                }
                              }
                              frame #2 {
                                # "Correct aberration"
                                n223 = stacked-sequence {
                                seq-local: [w381 _] -> [_ w526]
                                seq-local: [w380 _] -> [_ w525]
                                seq-local: [w379 _] -> [_ w523]
                                seq-local: [w378 _] -> [_ w524]
                                seq-local: [w377 _] -> [_ w527]
                                tunnel: w374 -> [w388 _]
                                tunnel: w373 -> [w387 _]
                                tunnel: w372 -> [w385 _]
                                tunnel: w371 -> [w384 _]
                                tunnel: w370 -> [w383 _]
                                tunnel: w369 -> [w382 _]
                                tunnel: w368 -> [w376 w522]
                                tunnel: [w375 _] -> w367
                                frame #0 {
                                n224 = for {
                                N: "Iteration #" -> [_]
                                tunnel: w388 -> [w420]
                                tunnel: w387 -> [w419]
                                tunnel: w385 -> [w418]
                                tunnel: w384 -> [w417]
                                tunnel: w383 -> [w416]
                                tunnel: [w414] -> w375
                                tunnel: w382 -> [w411]
                                tunnel: [w410] -> w381
                                tunnel: [w408] -> w380
                                tunnel: [w406] -> w379
                                tunnel: [w404] -> w378
                                tunnel: [w401] -> w377
                                tunnel: w376 -> [w400]
                                i -> [w399]
                                n225 = Increment(x=w399) -> (x+1=w398:i32)
                                n226 = flat-sequence {
                                tunnel: [w430] -> w425
                                tunnel: [w431] -> w424
                                tunnel: [w432] -> w423
                                tunnel: [w434] -> w422
                                tunnel: [w433] -> w421
                                tunnel: w420 -> [w434]
                                tunnel: w419 -> [w433]
                                tunnel: w418 -> [w432]
                                tunnel: w417 -> [w431]
                                tunnel: w416 -> [w430]
                                tunnel: [w429] -> w412
                                tunnel: w411 -> [w429]
                                tunnel: w398 -> [w427]
                                tunnel: [w426] -> w397
                                tunnel: w425 -> [w441]
                                tunnel: w424 -> [w442]
                                tunnel: w423 -> [w443]
                                tunnel: [w443] -> w395
                                tunnel: [w440] -> w394
                                tunnel: [w439] -> w393
                                tunnel: [w438] -> w392
                                tunnel: w422 -> [w438]
                                tunnel: [w437] -> w391
                                tunnel: w421 -> [w437]
                                tunnel: [w436] -> w390
                                tunnel: w412 -> [w436]
                                tunnel: [w435] -> w389
                                tunnel: w397 -> [w435]
                                tunnel: w393 -> [w502]
                                tunnel: w394 -> [w503]
                                tunnel: w395 -> [w504]
                                tunnel: w392 -> [w491]
                                tunnel: w391 -> [w490]
                                tunnel: [w471] -> w415
                                tunnel: [w470] -> w413
                                tunnel: w390 -> [w451]
                                tunnel: [w467] -> w409
                                tunnel: [w466] -> w407
                                tunnel: [w465] -> w405
                                tunnel: [w464] -> w403
                                tunnel: [w453] -> w402
                                tunnel: w400 -> [w450]
                                tunnel: w389 -> [w447]
                                tunnel: [w446] -> w396
                                tunnel: w415 -> [w516]
                                tunnel: [w515] -> w414
                                tunnel: w413 -> [w515]
                                tunnel: [w514] -> w410
                                tunnel: w409 -> [w514]
                                tunnel: [w513] -> w408
                                tunnel: w407 -> [w513]
                                tunnel: [w512] -> w406
                                tunnel: w405 -> [w512]
                                tunnel: [w508] -> w404
                                tunnel: w403 -> [w509]
                                tunnel: w402 -> [w511]
                                tunnel: [w511] -> w401
                                tunnel: w396 -> [w510]
                                frame #0 {
                                n227 = local read "Iteration #"() -> (w428:u16)
                                n228 = Less?(x=w428, y=w427) -> (x < y?=w426:bool)
                                }
                                frame #1 {
                                n229 = call "Camera Start.vi"("error in (no error)"=w441, "camera"=w442) -> ("error out"=w439:errorcluster, "camera (dup)"=w440:T3)  [unwired: 4 in]
                                }
                                frame #2 {
                                n230 = call "Camera Get image.vi"("error in (no error)"=w502, "camera"=w503) -> ("error out"=w487:errorcluster, "Image"=w488:T16, "camera (dup)"=w489:T3)  [unwired: 3 in]
                                n231 = call "Camera Stop.vi"("error in (no error)"=w487, "camera"=w489) -> ()  [unwired: 4 in, 2 out]
                                n232 = call "Image get data.vi"("error in (no error)"=w487, "Image Compat"=w488) -> ("error out"=w478:errorcluster, "Array"=w445:u32[][], "Image Compat (dup)"=w477:T16)  [unwired: 3 in]
                                n233 = local write "Camera image"(w445) -> ()
                                n234 = call "Haso compute slopes.vi"("error in (no error)"=w478, "Image Compat"=w477, "Haso"=w504) -> ("error out"=w456:errorcluster, "Data Haso"=w455:T12)  [unwired: 1 in, 2 out]
                                n235 = call "DataHaso get reconstruction prefs.vi"("error in (no error)"=w456, "Data Haso"=w455) -> ("error out"=w462:errorcluster, "Reconstruction Preferences"=w461:T19, "Data Haso (dup)"=w463:T12)  [unwired: 3 in]
                                n236 = Bundle By Name(cluster=w461, "Reconstruction type"=enum16{"Modal", "Zonal"}."Modal", "Polynomial type"=enum16{"Zernike", "Legendre"}."Zernike", "Modal reconstruction prefs.Number of coefficients"=u32 32) -> (w460:T19)
                                n237 = call "DataHaso set reconstruction prefs.vi"("error in (no error)"=w462, "Reconstruction Preferences"=w460, "Data Haso"=w463) -> ("error out"=w448:errorcluster, "Data Haso (dup)"=w449:T12)  [unwired: 3 in]
                                n238 = call "DataHaso get modal coefficients.vi"("error in (no error)"=w448, "Data Haso"=w449) -> ("error out"=w454:errorcluster, "Coefficients (µm)"=w453:sgl[], "Data Haso (dup)"=w452:T12)  [unwired: 3 in]
                                "Model Coefficients (µm) after" <- w453
                                n239 = call "DataHaso parameters.vi"("error in (no error)"=w454, "Data Haso"=w452) -> ("error out"=w485:errorcluster, "Parameters"=w465:T8, "Data Haso (dup)"=w486:T12)  [unwired: 3 in]
                                "after correction" <- w465
                                n240 = Bundle By Name(cluster=T11 {"Filtre tilt X"=FALSE, "Filtre tilt Y"=FALSE, "Filtre courbure"=FALSE} ("Filtre"), "Filtre tilt X"="Filter x tilt", "Filtre tilt Y"="Filter y tilt", "Filtre courbure"="Curvature filter") -> (w475:T11)
                                n241 = call "DataHaso filter tilt or curvature.vi"("error in (no error)"=w485, "Filter (default: all true)"=w475, "Data Haso"=w486) -> ("error out"=w483:errorcluster, "Data Haso (dup)"=w484:T12)  [unwired: 3 in]
                                n242 = call "DataHaso phase.vi"("error in (no error)"=w483, "Data Haso"=w484) -> ("error out"=w481:errorcluster, "Phase (µm)"=w482:i32, "Data Haso (dup)"=w469:T12)  [unwired: 3 in]
                                n243 = control-ref of="Wavefront after correction"() -> (w444:refnum<vi>)
                                n244 = call "Formatter Intensity Graph.vi"("error in (no error)"=w481, "Intensity Graph"=w444, "Surface with pupil"=w482) -> ("error out"=w479:errorcluster, "Surface with pupil (dup)"=w480:i32)  [unwired: 2 in, 1 out]
                                n245 = call "Surface with pupil get stats.vi"("error in (no error)"=w479, "Surface Avec Pupille"=w480) -> ("error out"=w497:errorcluster, "PV"=w466:sgl, "RMS"=w467:dbl)  [unwired: 2 in, 1 out]
                                "RMS" <- w467
                                "PV" <- w466
                                n246 = Merge Errors(w497, w490) -> (w496:errorcluster)
                                n247 = call "DataHaso ctor copie.vi"("error in (no error)"=w496, "DataHaso"=w469) -> ("error out"=w499:errorcluster, "new DataHaso"=w498:T12, "DataHaso (dup)"=w468:T12)  [unwired: 3 in]
                                n248 = Bundle By Name(cluster=T14 {"Target for tilt"=0, "Target for focus"=0, "Target for all other aberrations"=0} ("References"), "Target for tilt"=w450, "Target for focus"=w450) -> (w500:T14)
                                n249 = call "Casao Compute target.vi"("error in (no error)"=w499, "Targets"=w500, "DataHaso"=w498, "Casao"=w491) -> ("error out"=w494:errorcluster, "DataHaso (dup)"=w471:T12, "Casao (dup)"=w495:T6)  [unwired: 1 out]
                                n250 = Bundle By Name(cluster=T13 {"Measurement"=0, "Target"=0, "Manual target"=0} ("Slopes"), "Measurement"=w468, "Target"=w471) -> (w493:T13)
                                n251 = call "Casao get correction commands.vi"("Casao"=w495, "Slopes"=w493, "error in (no error)"=w494) -> ("Casao (dup)"=w470:T6, "Commands"=w464:sgl[], "error out"=w446:errorcluster)  [unwired: 2 in, 2 out]
                                n252 = case shown="True" w447 {
                                tunnel: w446 -> [_ w507]
                                tunnel: w464 -> [_ w506]
                                tunnel: w451 -> [_ w505]
                                frame False {
                                }
                                frame True {
                                n253 = call "PhaseModul apply command.vi"("error in (no error)"=w507, "Commands in"=w506, "Mirror"=w505) -> ()  [unwired: 2 in, 3 out]
                                }
                                }
                                }
                                frame #3 {
                                n254 = call "DataHaso dtor.vi"("Data Haso"=w516) -> ()  [unwired: 6 in, 1 out]
                                n255 = case shown="Error" w510 {
                                tunnel: w509 -> [w517 _]
                                tunnel: [w517 w518] -> w508
                                frame No Error {
                                }
                                frame Error {
                                n256 = Initialize Array(0.0 ("element"), 52 ("dimension size")) -> (w518:dbl[])
                                }
                                }
                                }
                                }
                                }
                                }
                                frame #1 {
                                n257 = call "DataHaso dtor.vi"("Data Haso"=w522) -> ()  [unwired: 6 in, 1 out]
                                n258 = local read "Slice now"() -> (w521:dbl)
                                n259 = Cluster To Array(cluster=w523) -> (array=w538:sgl[])
                                n260 = Build Array (concatenate)(w525, w526, w538, w527) -> (w536:dbl[])
                                n261 = Number To Decimal String(number=w521) -> (decimal integer string=w537:string)  [unwired: 1 in]
                                n262 = Number To Decimal String(number=w521) -> (decimal integer string=w539:string)  [unwired: 1 in]
                                n263 = local read "output path"() -> (w540:path)
                                n264 = Concatenate Strings("afterC_slice", w537, ".dat") -> (w541:string)
                                n265 = Concatenate Strings("command", w539, ".dat") -> (w543:string)
                                n266 = Build Path(base path=w540, name or relative path=w541) -> (appended path=w542:path)
                                n267 = Build Path(base path=w540, name or relative path=w543) -> (appended path=w544:path)
                                n268 = call-poly <vilib>:"Write To Spreadsheet File.vi"("transpose? (no:F)"=TRUE, "format (%.3f)"="%.6f", "1D data"=w536, "file path (dialog if empty)"=w542) -> ()  [unwired: 4 in, 1 out]
                                n269 = call-poly <vilib>:"Write To Spreadsheet File.vi"("transpose? (no:F)"=TRUE, "format (%.3f)"="%.6f", "1D data"=w524, "file path (dialog if empty)"=w544) -> ()  [unwired: 4 in, 1 out]
                                }
                                }
                              }
                              frame #3 {
                                # "Take image after AO correction"
                                n270 = stacked-sequence {
                                frame #0 {
                                n271 = local read "Flip Mirror Port"() -> (w545:tag)
                                n272 = Wait (ms)(milliseconds to wait=u32 100) -> ()  [unwired: 1 out]
                                n273 = call "AO single value.vi"("data"=-5.0, "physical channels"=w545) -> ()  [unwired: 1 in, 1 out]
                                }
                                frame #1 {
                                n274 = local read "Average Frame #"() -> (w548:dbl)
                                n275 = for {
                                N: w548 -> [_]
                                n276 = local read "stop"() -> (w549:bool)
                                n277 = Not(x=w549) -> (.not. x?=w550:bool)
                                n278 = case shown="False" w550 {
                                frame False {
                                }
                                frame True {
                                n279 = local read "ImExp Time (s)"() -> (w551:dbl)
                                n280 = local read "EMCCD trigger port"() -> (w552:tag)
                                n281 = Multiply(x=w551, y=1000.0) -> (x*y=w553:dbl)
                                n282 = call "trig EMCCD.vi"("exp time (ms)"=w553, "lines"=w552) -> ()  [unwired: 1 in, 1 out]
                                }
                                }
                                }
                                }
                                frame #2 {
                                # "Move Stage to next slice"
                                n283 = flat-sequence {
                                frame #0 {
                                n284 = local read "Step size(um)"() -> (w556:dbl)
                                n285 = Multiply(x=w556, y=10.0) -> (x*y=w559:dbl)
                                n286 = local read "Stage Port"() -> (w555:refnum<visa-resource-name>)
                                n287 = Number To Decimal String(number=w559) -> (decimal integer string=w561:string)  [unwired: 1 in]
                                n288 = Concatenate Strings("movrel z=", w561) -> (w560:string)
                                n289 = call "WriteCmd.vi"("Command"=w560, "VISA resource name"=w555) -> ()  [unwired: 1 in, 1 out]
                                }
                                frame #1 {
                                n290 = Wait (ms)(milliseconds to wait=u32 50) -> ()  [unwired: 1 out]
                                }
                                }
                                }
                                }
                              }
                            }
                          }
                        }
                      }
                    }
                    frame #2 {
                      n291 = call "Casao dtor.vi"("Casao"=w563) -> ()  [unwired: 6 in, 1 out]
                    }
                  }
                }
              }
            }
            frame #2 {
              n292 = local read "Step size(um)"() -> (w565:dbl)
              n293 = local read "Slices #"() -> (w566:dbl)
              n294 = Multiply(x=w565, y=-10.0) -> (x*y=w572:dbl)
              n295 = Multiply(x=w572, y=w566) -> (x*y=w571:dbl)
              n296 = Number To Decimal String(number=w571) -> (decimal integer string=w568:string)  [unwired: 1 in]
              n297 = Concatenate Strings("movrel z=", w568) -> (w569:string)
              n298 = call "AO single value.vi"("data"=0.0, "physical channels"=tag "Dev1/ao4") -> ()  [unwired: 1 in, 1 out]
              n299 = call "DO single value.vi"("data"=FALSE, "lines"=tag "Dev1/port0/line1") -> ()  [unwired: 1 in, 1 out]
              n300 = call "DO single value.vi"("data"=FALSE, "lines"=tag "Dev1/port0/line0") -> ()  [unwired: 1 in, 1 out]
              n301 = local read "Stage Port"() -> (w564:refnum<visa-resource-name>)
              n302 = call "WriteCmd.vi"("Command"=w569, "VISA resource name"=w564) -> ()  [unwired: 1 in, 1 out]
            }
          }
        }
        frame "Wide Field (Phase diversity)" {
          n303 = flat-sequence {
            tunnel: [w584] -> w581
            tunnel: [w583] -> w580
            tunnel: w581 -> [w590]
            tunnel: w580 -> [w589]
            tunnel: [w589] -> w579
            tunnel: w579 -> [w684]
            frame #0 {
              # "Initialize CASAO"
              n304 = call "Casao ctor.vi"("Mirror config file path"=path "C:/Program Files (x86)/Imagine Optic/Configuration Files/mirao 52-e 0225.xml", "Haso serial number"=u32 7364) -> ("error out"=w588:errorcluster, "Casao"=w587:T6)  [unwired: 6 in]
              n305 = call "Casao get PhaseModulator.vi"("error in (no error)"=w588, "Casao"=w587) -> ("error out"=w584:errorcluster, "Mirrror"=w583:T5, "Casao (dup)"=w582:T6)  [unwired: 3 in]
              n306 = local write "Casao Index"(w582) -> ()
            }
            frame #1 {
              n307 = stacked-sequence {
                tunnel: w590 -> [w593 w610 w629 w648 w667]
                tunnel: w589 -> [w592 w609 w628 w647 w666]
                frame #0 {
                  n308 = flat-sequence {
                    tunnel: w593 -> [w600]
                    tunnel: w592 -> [w597]
                    tunnel: [w595] -> w591
                    tunnel: w591 -> [w602]
                    frame #0 {
                      n309 = local read "Phase command 0"() -> (w596:path)
                      n310 = call-poly <vilib>:"Read From Spreadsheet File.vi"("format (%.3f)"="%.8f", "file path (dialog if empty)"=w596) -> ("first row"=w598:dbl[])  [unwired: 5 in, 4 out]
                      n311 = call "PhaseModul apply command.vi"("error in (no error)"=w600, "Commands in"=w598, "Mirror"=w597) -> ("error out"=w595:errorcluster)  [unwired: 2 in, 2 out]
                      n312 = Wait (ms)(milliseconds to wait=100) -> ()  [unwired: 1 out]
                    }
                    frame #1 {
                      n313 = local read "Average Frame #"() -> (w601:dbl)
                      n314 = for {
                        N: w601 -> [_]
                        tunnel: w602 -> [w603]
                        n315 = local read "EMCCD trigger port"() -> (w606:tag)
                        n316 = local read "ImExp Time (s)"() -> (w607:dbl)
                        n317 = Multiply(x=w607, y=1000.0) -> (x*y=w605:dbl)
                        n318 = call "trig EMCCD.vi"("error in (no error)"=w603, "exp time (ms)"=w605, "lines"=w606) -> ()  [unwired: 1 out]
                      }
                    }
                  }
                }
                frame #1 {
                  n319 = flat-sequence {
                    tunnel: w610 -> [w617]
                    tunnel: w609 -> [w611]
                    tunnel: [w613] -> w608
                    tunnel: w608 -> [w620]
                    tunnel: [w618] -> _
                    frame #0 {
                      n320 = local read "Phase command 1"() -> (w614:path)
                      n321 = call-poly <vilib>:"Read From Spreadsheet File.vi"("format (%.3f)"="%.8f", "file path (dialog if empty)"=w614) -> ("first row"=w615:dbl[])  [unwired: 5 in, 4 out]
                      n322 = call "PhaseModul apply command.vi"("error in (no error)"=w617, "Commands in"=w615, "Mirror"=w611) -> ("error out"=w613:errorcluster)  [unwired: 2 in, 2 out]
                      n323 = Wait (ms)(milliseconds to wait=100) -> ()  [unwired: 1 out]
                    }
                    frame #1 {
                      n324 = local read "Average Frame #"() -> (w619:dbl)
                      n325 = for {
                        N: w619 -> [_]
                        tunnel: w620 -> [w622]
                        tunnel: [w621] -> w618 mode=indexing
                        n326 = local read "EMCCD trigger port"() -> (w625:tag)
                        n327 = local read "ImExp Time (s)"() -> (w626:dbl)
                        n328 = Multiply(x=w626, y=1000.0) -> (x*y=w624:dbl)
                        n329 = call "trig EMCCD.vi"("error in (no error)"=w622, "exp time (ms)"=w624, "lines"=w625) -> ("error out"=w621:errorcluster)
                      }
                    }
                  }
                }
                frame #2 {
                  n330 = flat-sequence {
                    tunnel: w629 -> [w636]
                    tunnel: w628 -> [w630]
                    tunnel: [w632] -> w627
                    tunnel: w627 -> [w639]
                    tunnel: [w637] -> _
                    frame #0 {
                      n331 = local read "Phase command 2"() -> (w633:path)
                      n332 = call-poly <vilib>:"Read From Spreadsheet File.vi"("format (%.3f)"="%.8f", "file path (dialog if empty)"=w633) -> ("first row"=w634:dbl[])  [unwired: 5 in, 4 out]
                      n333 = call "PhaseModul apply command.vi"("error in (no error)"=w636, "Commands in"=w634, "Mirror"=w630) -> ("error out"=w632:errorcluster)  [unwired: 2 in, 2 out]
                      n334 = Wait (ms)(milliseconds to wait=100) -> ()  [unwired: 1 out]
                    }
                    frame #1 {
                      n335 = local read "Average Frame #"() -> (w638:dbl)
                      n336 = for {
                        N: w638 -> [_]
                        tunnel: w639 -> [w641]
                        tunnel: [w640] -> w637 mode=indexing
                        n337 = local read "EMCCD trigger port"() -> (w644:tag)
                        n338 = local read "ImExp Time (s)"() -> (w645:dbl)
                        n339 = Multiply(x=w645, y=1000.0) -> (x*y=w643:dbl)
                        n340 = call "trig EMCCD.vi"("error in (no error)"=w641, "exp time (ms)"=w643, "lines"=w644) -> ("error out"=w640:errorcluster)
                      }
                    }
                  }
                }
                frame #3 {
                  n341 = flat-sequence {
                    tunnel: w648 -> [w655]
                    tunnel: w647 -> [w649]
                    tunnel: [w651] -> w646
                    tunnel: w646 -> [w658]
                    tunnel: [w656] -> _
                    frame #0 {
                      n342 = local read "Phase command 3"() -> (w652:path)
                      n343 = call-poly <vilib>:"Read From Spreadsheet File.vi"("format (%.3f)"="%.8f", "file path (dialog if empty)"=w652) -> ("first row"=w653:dbl[])  [unwired: 5 in, 4 out]
                      n344 = call "PhaseModul apply command.vi"("error in (no error)"=w655, "Commands in"=w653, "Mirror"=w649) -> ("error out"=w651:errorcluster)  [unwired: 2 in, 2 out]
                      n345 = Wait (ms)(milliseconds to wait=100) -> ()  [unwired: 1 out]
                    }
                    frame #1 {
                      n346 = local read "Average Frame #"() -> (w657:dbl)
                      n347 = for {
                        N: w657 -> [_]
                        tunnel: w658 -> [w660]
                        tunnel: [w659] -> w656 mode=indexing
                        n348 = local read "EMCCD trigger port"() -> (w663:tag)
                        n349 = local read "ImExp Time (s)"() -> (w664:dbl)
                        n350 = Multiply(x=w664, y=1000.0) -> (x*y=w662:dbl)
                        n351 = call "trig EMCCD.vi"("error in (no error)"=w660, "exp time (ms)"=w662, "lines"=w663) -> ("error out"=w659:errorcluster)
                      }
                    }
                  }
                }
                frame #4 {
                  n352 = flat-sequence {
                    tunnel: w667 -> [w674]
                    tunnel: w666 -> [w668]
                    tunnel: [w670] -> w665
                    tunnel: w665 -> [w677]
                    tunnel: [w675] -> _
                    frame #0 {
                      n353 = local read "Phase command 0"() -> (w671:path)
                      n354 = call-poly <vilib>:"Read From Spreadsheet File.vi"("format (%.3f)"="%.8f", "file path (dialog if empty)"=w671) -> ("first row"=w672:dbl[])  [unwired: 5 in, 4 out]
                      n355 = call "PhaseModul apply command.vi"("error in (no error)"=w674, "Commands in"=w672, "Mirror"=w668) -> ("error out"=w670:errorcluster)  [unwired: 2 in, 2 out]
                      n356 = Wait (ms)(milliseconds to wait=100) -> ()  [unwired: 1 out]
                    }
                    frame #1 {
                      n357 = local read "Average Frame #"() -> (w676:dbl)
                      n358 = for {
                        N: w676 -> [_]
                        tunnel: w677 -> [w679]
                        tunnel: [w678] -> w675 mode=indexing
                        n359 = local read "EMCCD trigger port"() -> (w682:tag)
                        n360 = local read "ImExp Time (s)"() -> (w683:dbl)
                        n361 = Multiply(x=w683, y=1000.0) -> (x*y=w681:dbl)
                        n362 = call "trig EMCCD.vi"("error in (no error)"=w679, "exp time (ms)"=w681, "lines"=w682) -> ("error out"=w678:errorcluster)
                      }
                    }
                  }
                }
              }
            }
            frame #2 {
              n363 = call "Casao dtor.vi"("Casao"=w684) -> ()  [unwired: 6 in, 1 out]
            }
          }
        }
      }
    }
    frame "Shut Down" {
      n364 = local read "Casao Index"() -> (w686:T6)
      n365 = call "Casao dtor.vi"("Casao"=w686) -> ("error out"=w685:errorcluster)  [unwired: 6 in]
      "Shutdown error" <- w685
      n366 = local write "Initialization error"(w685) -> ()
    }
  }
